vi "ex04_basic_data_types.vi"() -> ()   [LabVIEW 2019]
panel:
  out "Meter 3":u8(knob) scale=0.0..10.0
  out "Meter 2":u8(knob) scale=0.0..10.0
  in  "Knob 2":u8(knob) scale=0.0..10.0
  out "Meter":dbl(knob) scale=0.0..10.0
  in  "Knob":dbl(knob) scale=0.0..10.0
  out "Boolean 3":bool
  in  "Boolean 2":bool
  out "String":string="LabVIEW"
  out "Numeric 5":dbl=3.141592653589793
  out "Numeric 4":dbl=2.220446049250313e-16
  out "Numeric 2":dbl=3.14
  out "Numeric":i32=123
  out "Boolean":bool=TRUE
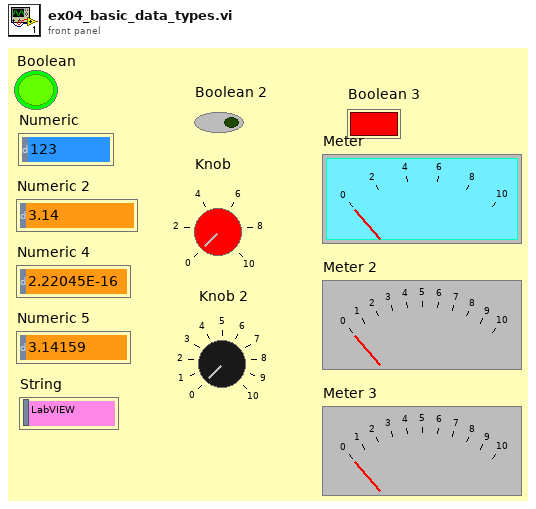
[diagram p1: front panel]
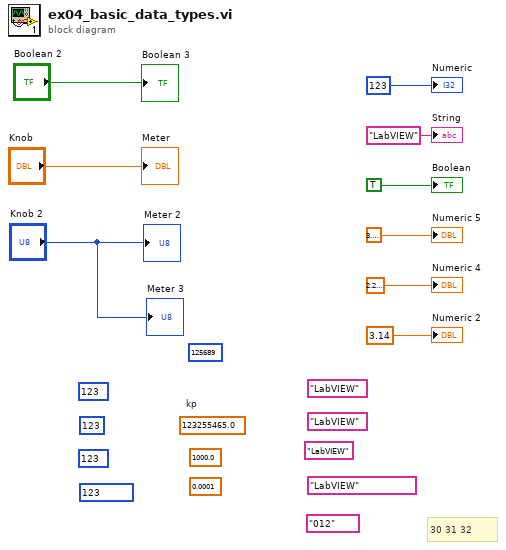
[diagram p0: block diagram]
diagram:
  (unwired) "012"
  (unwired) "LabVIEW"
  (unwired) "LabVIEW"
  (unwired) "LabVIEW"
  (unwired) "LabVIEW"
  (unwired) 0.0001
  (unwired) 1000.0
  (unwired) 123255465.0  # kp
  (unwired) 125689
  (unwired) 123 ("Speed")
  (unwired) 123 ("Speed")
  (unwired) 123 ("Speed")
  (unwired) 123 ("Speed")
  # "30 31 32"
  "Boolean" <- TRUE
  "Numeric" <- 123
  "Numeric 2" <- 3.14
  "Numeric 4" <- 2.220446049250313e-16
  "Numeric 5" <- 3.141592653589793
  "String" <- "LabVIEW"
  "Boolean 3" <- "Boolean 2"
  "Meter" <- "Knob"
  "Meter 2" <- "Knob 2"
  "Meter 3" <- "Knob 2"
